vi "Write layout.vi"(8 "error in (no error)":errorcluster, 10 "Lumberjack.lvlib:Layout.lvclass":refnum<class "Layout.lvclass">, 11 "FileAppender in":refnum<class "FileAppender.lvclass">) -> (0 "error out":errorcluster, 3 "FileAppender out":refnum<class "FileAppender.lvclass">)   [LabVIEW 2026, in "Lumberjack.lvlib" / "FileAppender.lvclass"]
doc: "Stores the Layout object into the file appender's private data.\nClass private-data accessor; sets the layout used when writing lines to the file. No side effects.\nLumberjack.lvlib, FileAppender.lvclass, protected."
uses:
  FileAppender.lvclass
  Layouts/Layout.lvclass/Layout.lvclass
  FileAppender.lvclass/FileAppender.ctl
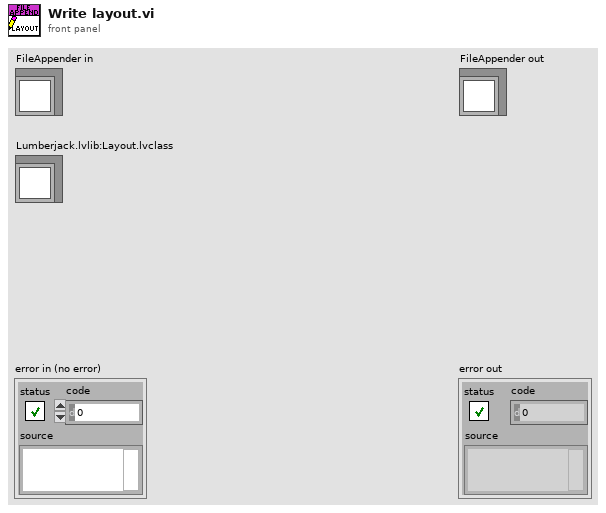
[diagram p1: front panel]
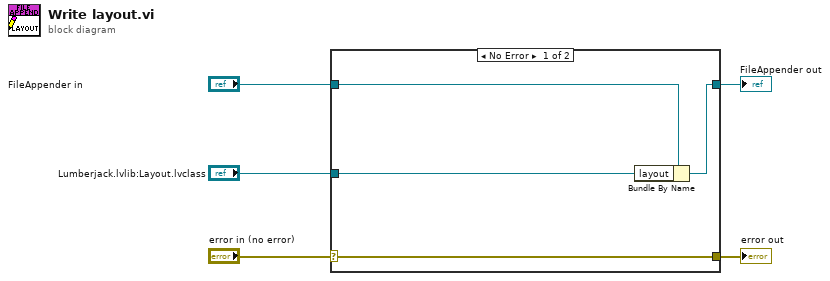
[diagram p0: block diagram]
diagram:
  n1 = case shown="No Error" "error in (no error)" {
    selector: "error in (no error)" -> [w9 w10]
    tunnel: [w9 w10] -> w4
    tunnel: [w7 w11] -> w2
    tunnel: "FileAppender in" -> [w8 w11]
    tunnel: "Lumberjack.lvlib:Layout.lvclass" -> [w6 _]
    frame No Error {
      n2 = Bundle By Name(cluster=w8, "layout"=w6) -> (w7:refnum<class "FileAppender.lvclass">)
    }
    frame Error {
    }
  }
  "error out" <- w4
  "FileAppender out" <- w2
